vi "SSCP_test.vi"() -> ()   [LabVIEW 2020]
uses:
  sscp/typedefs/Device Configuration.ctl
  sscp/commands.ctl
panel:
  out "Button 1 press count":dbl
  out "Button 0 press count":dbl
  in  "Device Configuration":T1={"Device name"="default", "Device number"="0", "Serial Port"="COM9", "Serial baud rate"="115200", "Base Port"="3000", "Device Serial Number"="1", "Interface Timeout"="10000", "Interface Type"="SERIAL"}
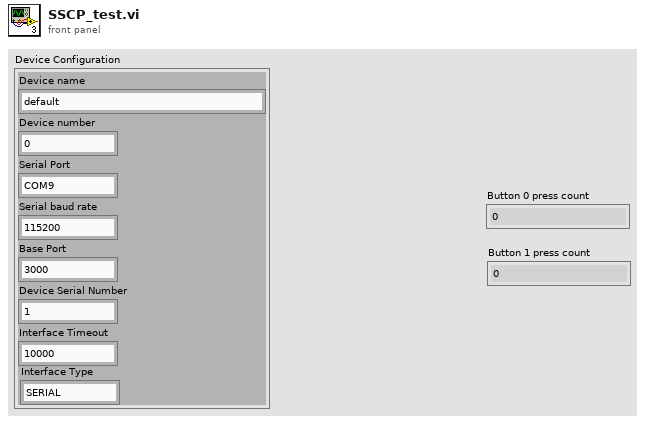
[diagram p1: front panel]
types:
  T1 = typedef "Device Configuration.ctl" = cluster{"Device name":string, "Device number":string, "Serial Port":string, "Serial baud rate":string, "Base Port":string, "Device Serial Number":string, "Interface Timeout":string, "Interface Type":string}
  T2 = typedef "commands.ctl" = enum16{"INIT", "CONFIGURE", "CONNECT", "GET_PARAMETER", "GET_PARAMETER_FROM_DEVICE", "SET_PARAMETER", "SET_PARAMETER_IN_DEVICE", "READ_REGISTER", "WRITE_REGISTER", "DISCONNECT"}
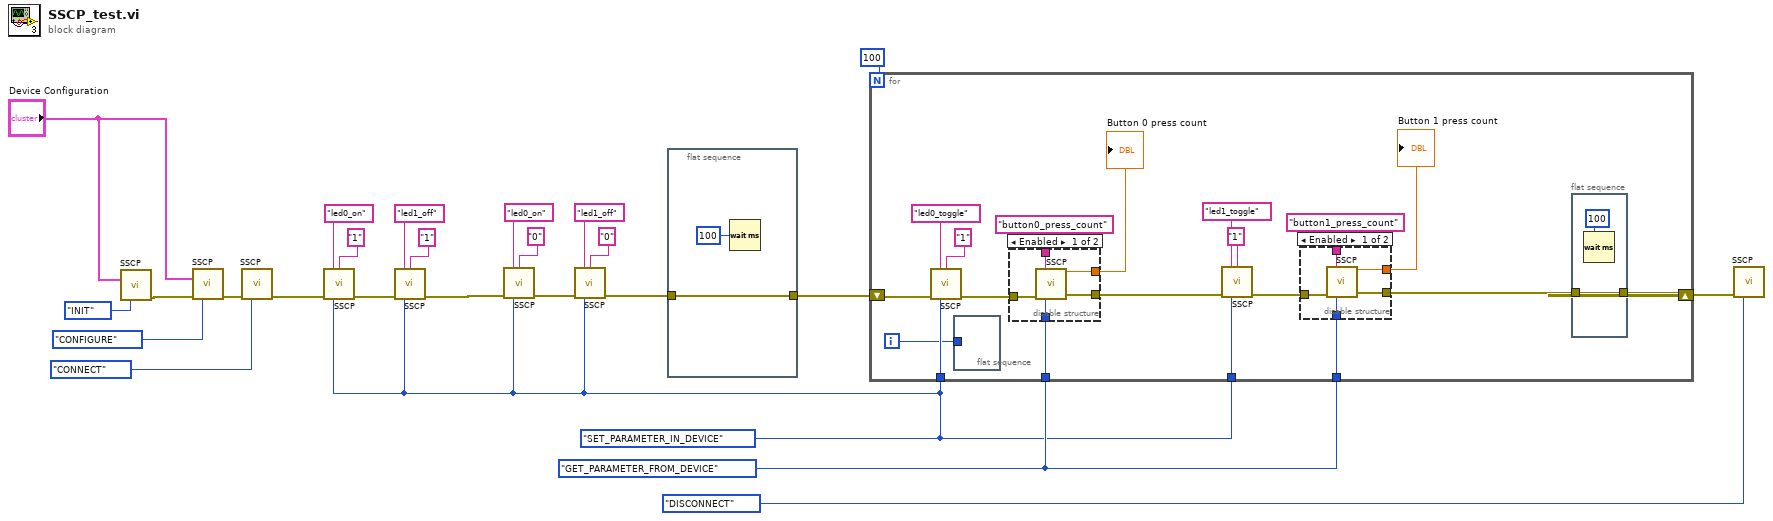
[diagram p0: block diagram]
diagram:
  w16 = commands."GET_PARAMETER_FROM_DEVICE" ("Command")
  w3 = commands."SET_PARAMETER_IN_DEVICE" ("Command")
  n1 = call "SSCP.vi"("Device Configuration"="Device Configuration", "Command"=commands."INIT") -> ("error out"=w24:errorcluster)  [unwired: 12 in, 1 out]
  n2 = call "SSCP.vi"("Device Configuration"="Device Configuration", "error in (no error)"=w24, "Command"=commands."CONFIGURE") -> ("error out"=w18:errorcluster)  [unwired: 11 in, 1 out]
  n3 = call "SSCP.vi"("error in (no error)"=w18, "Command"=commands."CONNECT") -> ("error out"=w13:errorcluster)  [unwired: 12 in, 1 out]
  n4 = call "SSCP.vi"("Parameter name"="led0_on", "Parameter value"="1", "error in (no error)"=w13, "Command"=w3) -> ("error out"=w10:errorcluster)  [unwired: 10 in, 1 out]
  n5 = call "SSCP.vi"("Parameter name"="led1_off", "Parameter value"="1", "error in (no error)"=w10, "Command"=w3) -> ("error out"=w4:errorcluster)  [unwired: 10 in, 1 out]
  n6 = call "SSCP.vi"("Parameter name"="led0_on", "Parameter value"="0", "error in (no error)"=w4, "Command"=w3) -> ("error out"=w5:errorcluster)  [unwired: 10 in, 1 out]
  n7 = call "SSCP.vi"("Parameter name"="led1_off", "Parameter value"="0", "error in (no error)"=w5, "Command"=w3) -> ("error out"=w2:errorcluster)  [unwired: 10 in, 1 out]
  n8 = flat-sequence {
    tunnel: w2 -> [w27]
    tunnel: [w27] -> w1
    frame #0 {
      n9 = Wait (ms)(milliseconds to wait=u32 100) -> ()  [unwired: 1 out]
    }
  }
  n10 = for {
    N: 100 -> [_]
    tunnel: w3 -> [w46]
    tunnel: w16 -> [w40]
    shift-right: [w29] -> w21
    shift-left: w1 -> [w39]
    tunnel: w3 -> [w32]
    tunnel: w16 -> [w31]
    i -> [w28]
    n11 = call "SSCP.vi"("Parameter name"="led0_toggle", "Parameter value"="1", "error in (no error)"=w39, "Command"=w46) -> ("error out"=w43:errorcluster)  [unwired: 10 in, 1 out]
    n12 = flat-sequence {
      tunnel: w28 -> [_]
      frame #0 {
      }
    }
    n13 = disable-structure shown="Enabled" {
      disable-tunnel: w43 -> [w59 w60]
      disable-tunnel: "button0_press_count" ("Parameter name") -> [w58 _]
      disable-tunnel: [w57 _] -> w41
      disable-tunnel: w40 -> [w56 _]
      disable-tunnel: [w55 w60] -> w33
      frame Enabled {
        n14 = call "SSCP.vi"("Parameter name"=w58, "error in (no error)"=w59, "Command"=w56) -> ("Parameter value"=w57:dbl, "error out"=w55:errorcluster)  [unwired: 11 in]
      }
      frame Disabled {
      }
    }
    "Button 0 press count" <- w41
    n15 = call "SSCP.vi"("Parameter name"="led1_toggle", "Parameter value"="1", "error in (no error)"=w33, "Command"=w32) -> ("error out"=w36:errorcluster)  [unwired: 10 in, 1 out]
    n16 = disable-structure shown="Enabled" {
      disable-tunnel: w36 -> [w51 w52]
      disable-tunnel: "button1_press_count" ("Parameter name") -> [w50 _]
      disable-tunnel: [w49 _] -> w34
      disable-tunnel: [w48 w52] -> w30
      disable-tunnel: w31 -> [w47 _]
      frame Enabled {
        n17 = call "SSCP.vi"("Parameter name"=w50, "error in (no error)"=w51, "Command"=w47) -> ("Parameter value"=w49:dbl, "error out"=w48:errorcluster)  [unwired: 11 in]
      }
      frame Disabled {
      }
    }
    "Button 1 press count" <- w34
    n18 = flat-sequence {
      tunnel: w30 -> [w53]
      tunnel: [w53] -> w29
      frame #0 {
        n19 = Wait (ms)(milliseconds to wait=u32 100) -> ()  [unwired: 1 out]
      }
    }
  }
  n20 = call "SSCP.vi"("error in (no error)"=w21, "Command"=commands."DISCONNECT") -> ()  [unwired: 12 in, 2 out]
